vi "SETTINGS.vi"() -> ()   [LabVIEW 2021]
uses:
  Control 1.ctl
  ENNUM CONSTANT.ctl
  Control 4.ctl
  <vilib>/Utility/miscctls.llb/LVPointTypeDef.ctl
  SETTING CLOSE GLOBEL VARIABLE.vi
  <vilib>/Utility/config.llb/Write Key (String).vi
  <vilib>/Utility/config.llb/Write Key (Double).vi
  <vilib>/Utility/config.llb/NI_LVConfig.lvlib
panel:
  in  "Copy to alll":bool
  in  "ENTER":bool
  in  "PASS KEY":string
  in  "TIME DELAY":dbl
  in  "RETEST":bool
  out "String":string
  in  "VISA resource name":refnum<visa-resource-name>="COM5"
  in  "SAVE":bool
  in  "TOL 10":dbl
  in  "CH 10":dbl
  in  "TOL 9":dbl
  in  "CH 9":dbl
  in  "TOL 8":dbl
  in  "CH 8":dbl
  in  "TOL 7":dbl
  in  "CH 7":dbl
  in  "TOL 6":dbl
  in  "CH 6":dbl
  in  "TOL 5":dbl
  in  "CH 5":dbl
  in  "TOL 4":dbl
  in  "CH 4":dbl
  in  "TOL 3":dbl
  in  "CH 3":dbl
  in  "TOL 2":dbl
  in  "CH 2":dbl
  in  "TOL 1":dbl
  in  "CH 1":dbl
  in  "Combo Box":string(combo)
  in  "Home 2":T1
  # "EOL TEST BENCH FOR THERMISTOR"
  # "NOMINAL & TOLERANCE VALUES"
  # "MODE"
  # "DEVICE CONFIGURATION"
  # "k Ohm"
  # "Channel 1"
  # "%"
  # "REFERENCE RESISTANCE VALUE (CH 5)"
  # "COM PORT"
  # "k Ohm"
  # "Channel 2"
  # "%"
  # "k Ohm"
  # "Channel 3"
  # "k Ohm"
  # "%"
  # "Channel 4"
  # "k Ohm"
  # "%"
  # "Channel 5"
  # "k Ohm"
  # "%"
  # "THERMAL TIME DELAY"
  # "k Ohm"
  # "Channel 6"
  # "%"
  # "Sec"
  # "RETEST"
  # "k Ohm"
  # "Channel 7"
  # "%"
  # "k Ohm"
  # "Channel 8"
  # "%"
  # "AUTHENTICATION KEY"
  # "Channel 9"
  # "k Ohm"
  # "%"
  # "k Ohm"
  # "Channel 10"
  # "%"
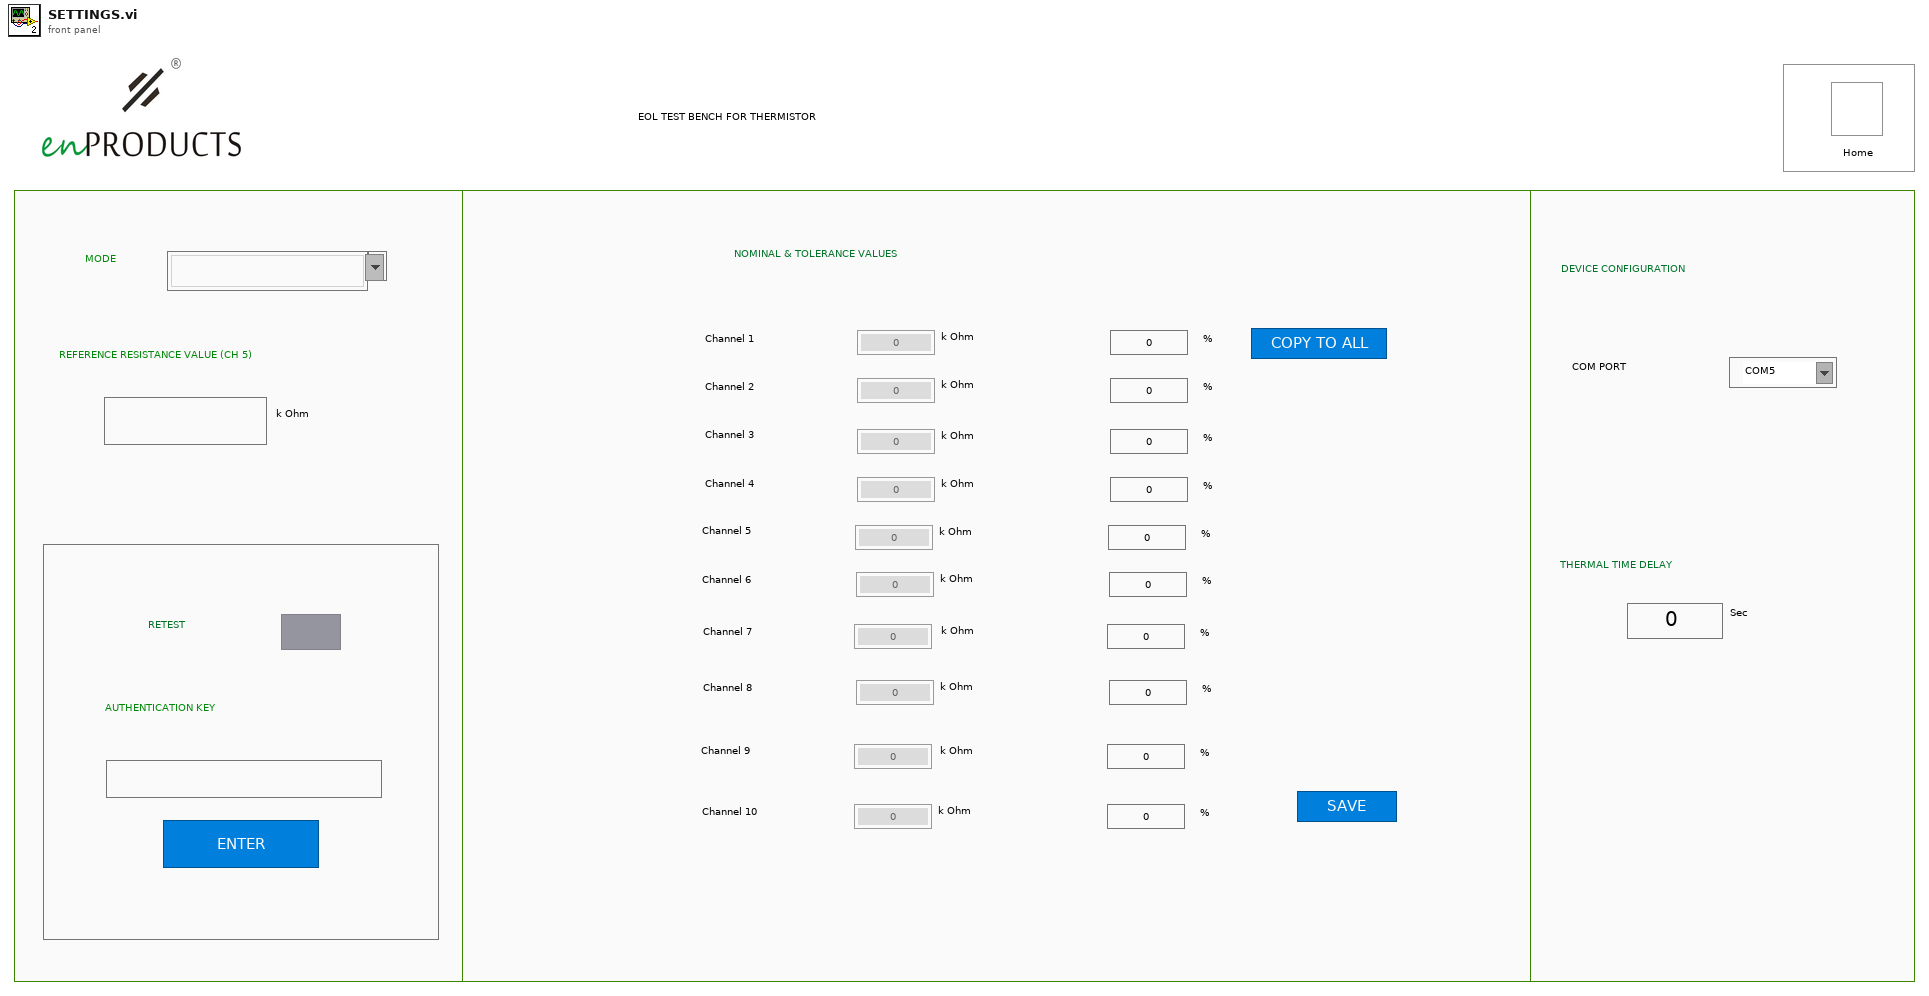
[diagram p1: front panel]
types:
  T1 = typedef "Control 1.ctl" = bool
  T2 = typedef "LVPointTypeDef.ctl" = cluster{"Horizontal":i16, "Vertical":i16}
  T3 = typedef "Control 4.ctl" = cluster{"VISA resource name":refnum<visa-resource-name>, "MODE":string, "PP 1":i32, "PP 2":i32, "PP 3":i32, "PP 4":i32, "PP 5":i32, "PP 6":i32, "PP 7":i32, "PP 8":i32, "PP 9":i32, "PP 10":i32, "CH  PASS  1":bool, "CH  PASS 2":bool, "CH  PASS 3":bool, "CH  PASS 4":bool, "CH  PASS 5":bool, "CH  PASS 6":bool, "CH  PASS 7":bool, "CH  PASS 8":bool, "CH  PASS 9":bool, "CH  PASS 10":bool, "CH  FAIL 1":bool, "CH  FAIL 2":bool, "CH  FAIL 3":bool, "CH  FAIL 4":bool, "CH  FAIL 5":bool, "CH  FAIL 6":bool, "CH  FAIL 7":bool, "CH  FAIL 8":bool, "CH  FAIL 9":bool, "CH  FAIL 10":bool, "RES VALUE 1":dbl, "RES VALUE 2":dbl, "RES VALUE 3":dbl, "RES VALUE 4":dbl, "RES VALUE 5":dbl, "RES VALUE 6":dbl, "RES VALUE 7":dbl, "RES VALUE 8":dbl, "RES VALUE 9":dbl, "RES VALUE 10":dbl, "SET VALUE 1":dbl, "SET VALUE 2":dbl, "SET VALUE 3":dbl, "SET VALUE 4":dbl, "SET VALUE 5":dbl, "SET VALUE 6":dbl, "SET VALUE 7":dbl, "SET VALUE 8":dbl, "SET VALUE 9":dbl, "SET VALUE 10":dbl, "TOL 1":dbl, "TOL 2":dbl, "TOL 3":dbl, "TOL 4":dbl, "TOL 5":dbl, "TOL 6":dbl, "TOL 7":dbl, "TOL 8":dbl, "TOL 9":dbl, "TOL 10":dbl, "START BIT":i32, "CH1 MIN TOL":dbl, "CH2 MIN TOL ":dbl, "CH3 MIN TOL ":dbl, "CH4 MIN TOL ":dbl, "CH5 MIN TOL ":dbl, "CH6 MIN TOL ":dbl, "CH7 MIN TOL  ":dbl, "CH8 MIN TOL  ":dbl, "CH9 MIN TOL   ":dbl, "CH10 MIN TOL   ":dbl, "CH1 MAX TOL ":dbl, "CH2 MAX TOL  ":dbl, "CH3 MAX TOL  ":dbl, "CH4 MAX TOL ":dbl, "CH5 MAX TOL  ":dbl, "CH6 MAX TOL  ":dbl, "CH7 MAX TOL   ":dbl, "CH8 MAX TOL  ":dbl, "CH9 MAX TOL    ":dbl, "CH10 MAX TOL   ":dbl}
  T4 = typedef "ENNUM CONSTANT.ctl" = enum16{"TIMEOUT", "INITIALIZE", "CONFIG READ", "CONFIG WRITE"}
  T5 = enum8{"Enabled", "Disabled", "Disabled and Grayed Out"}
  T6 = typedef "NI_LVConfig.lvlib/Config Data RefNum.ctl" = refnum<k1>
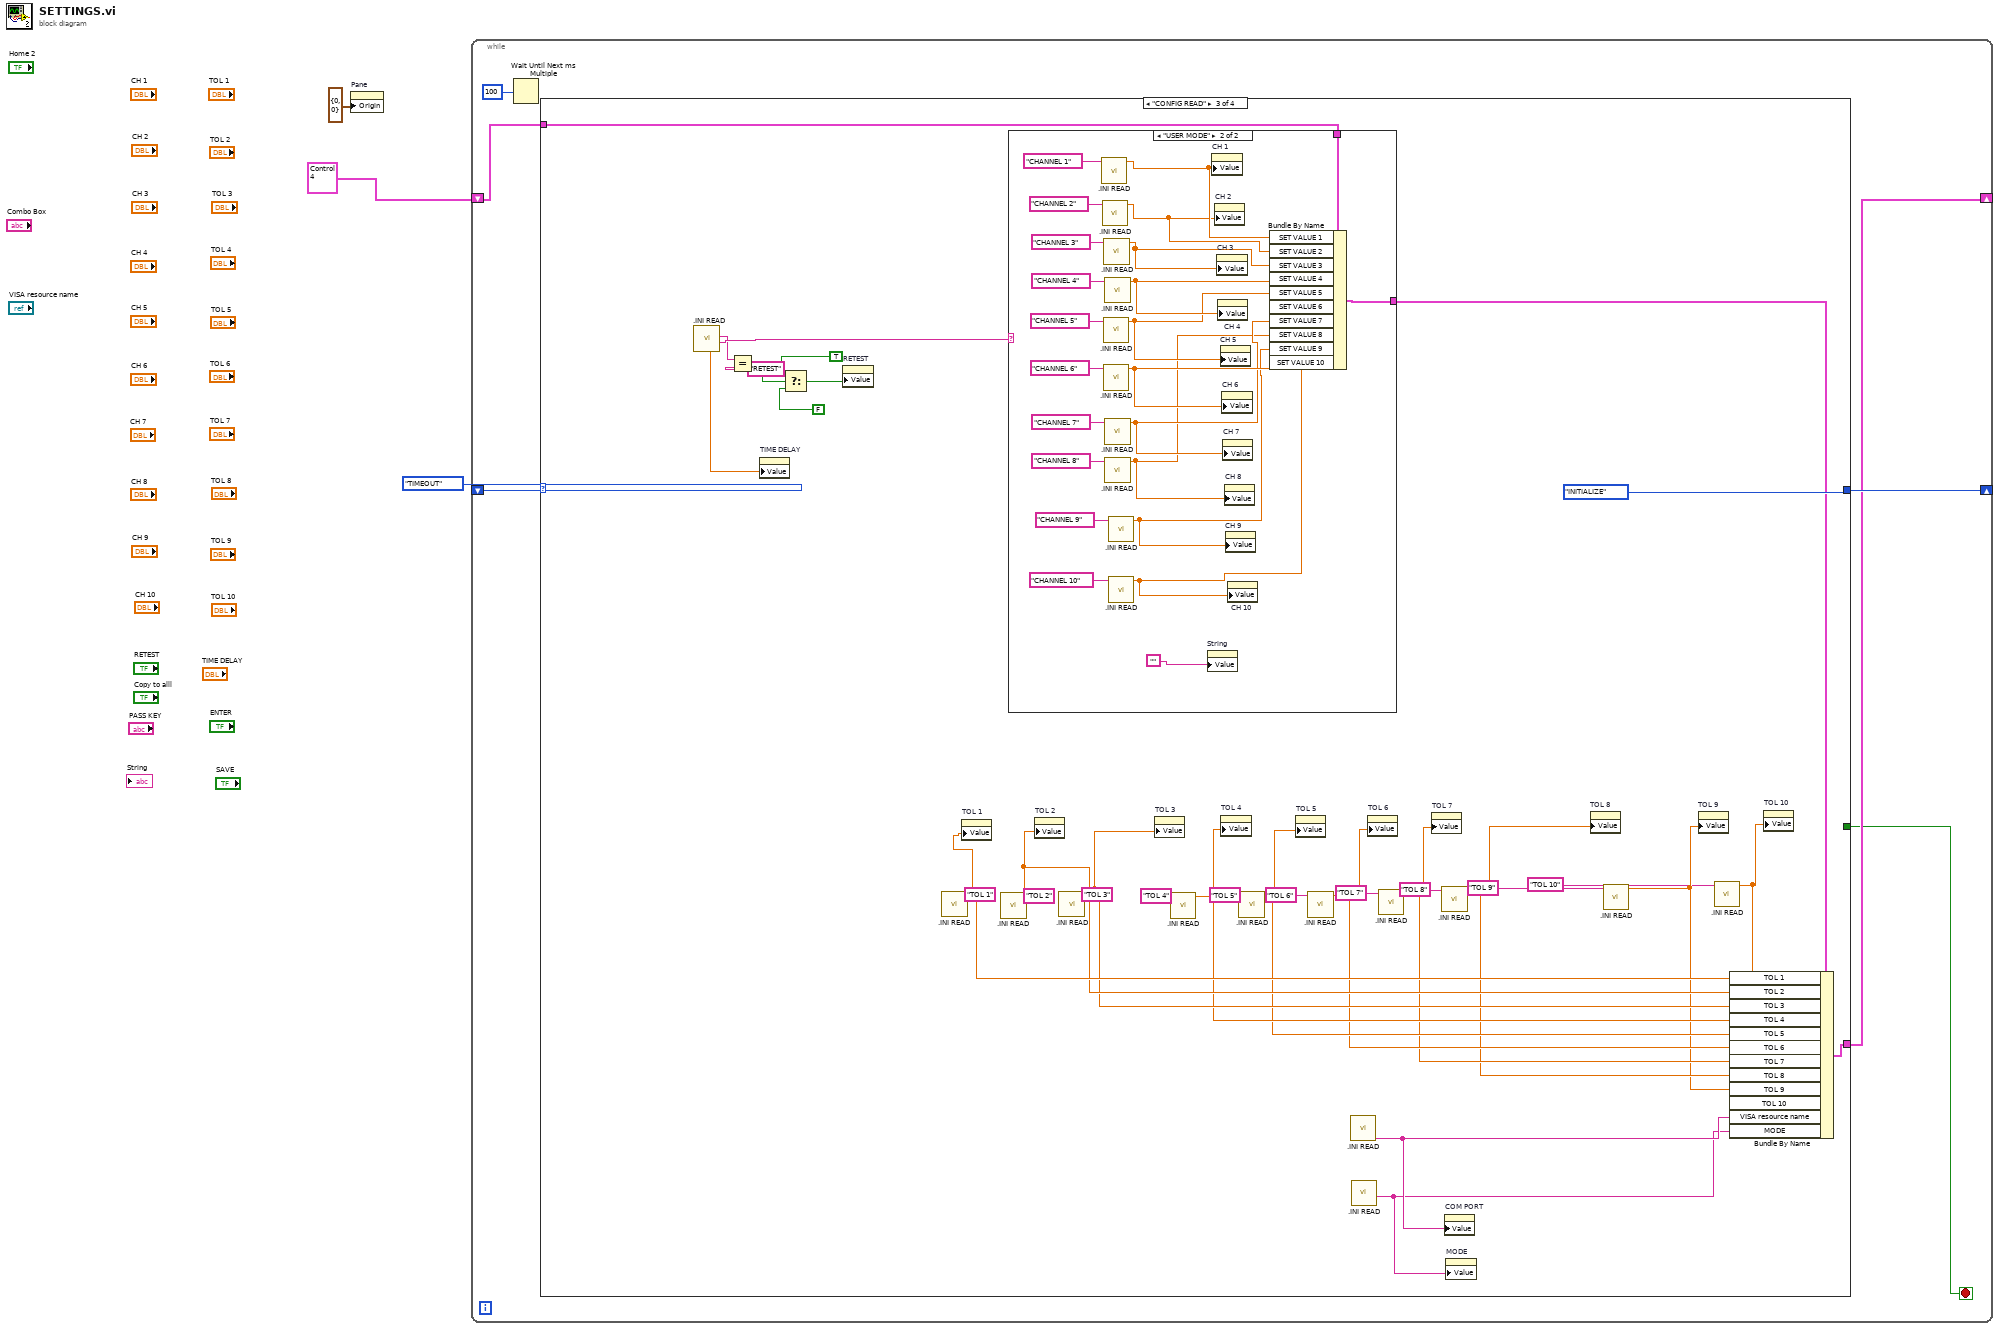
[diagram p0: block diagram]
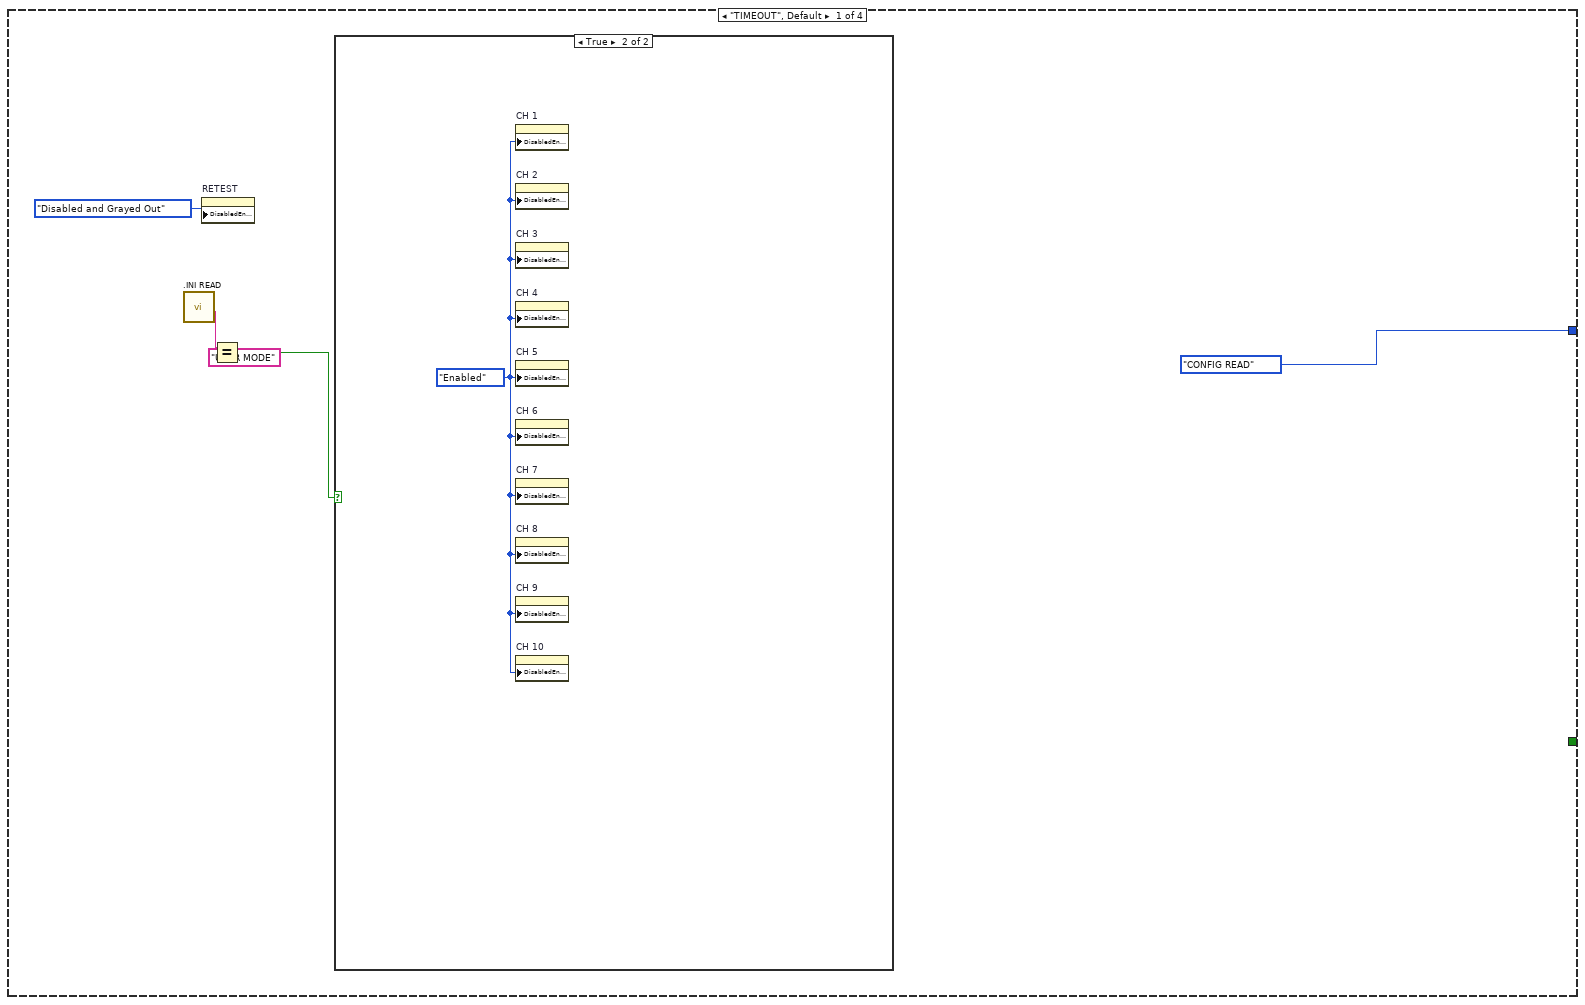
[diagram p2: hidden frame]
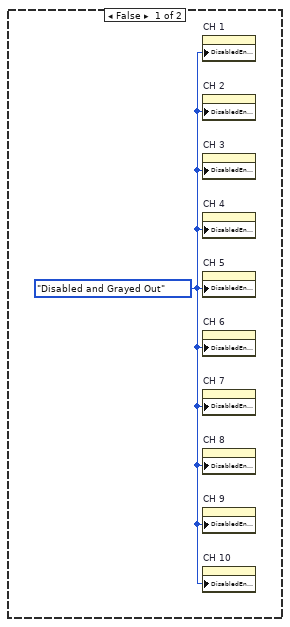
[diagram p3: hidden frame]
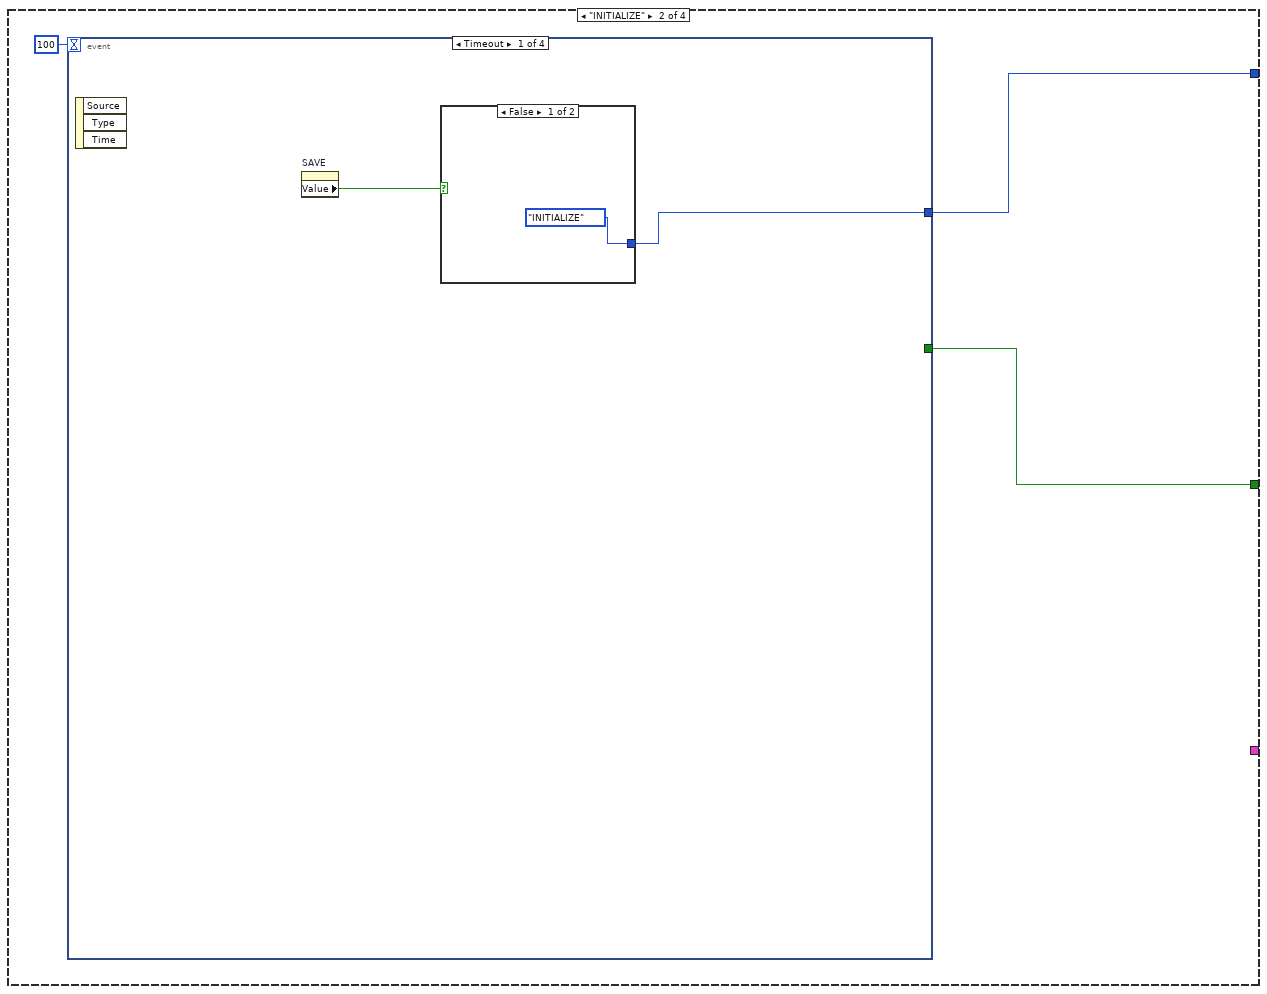
[diagram p4: hidden frame]
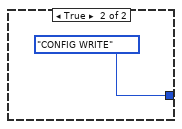
[diagram p5: hidden frame]
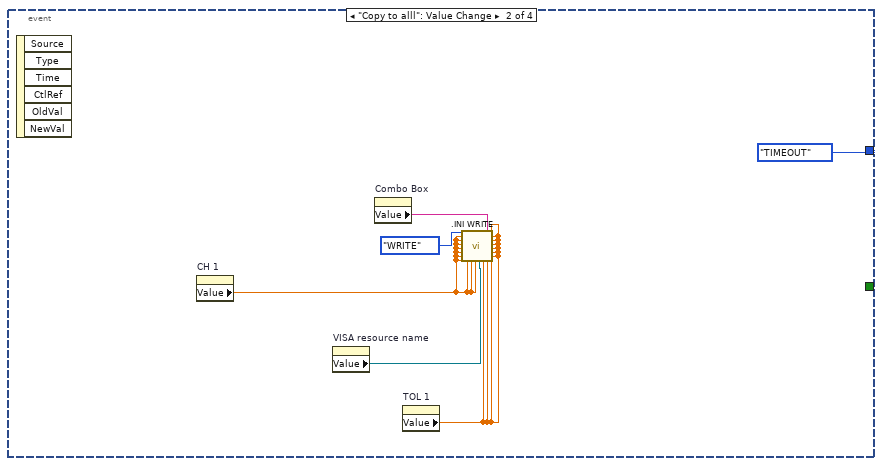
[diagram p6: hidden frame]
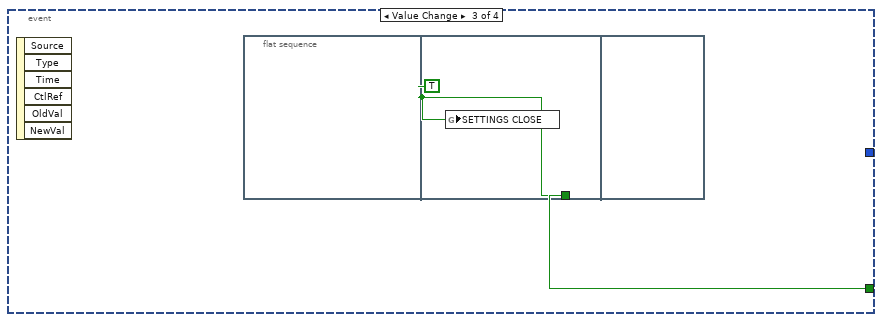
[diagram p7: hidden frame]
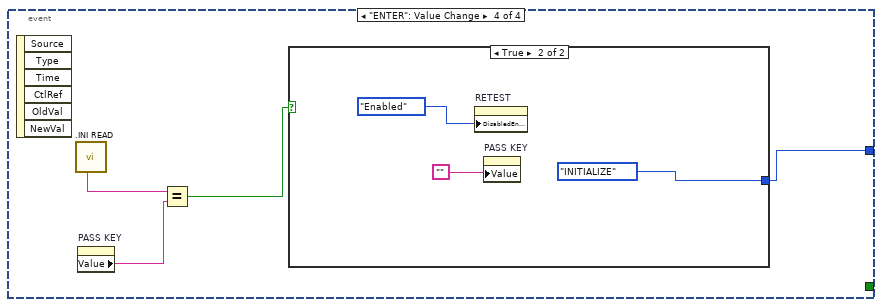
[diagram p8: hidden frame]
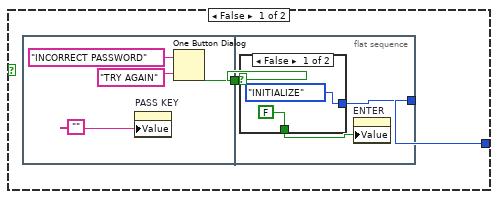
[diagram p9: hidden frame]
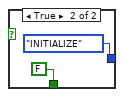
[diagram p10: hidden frame]
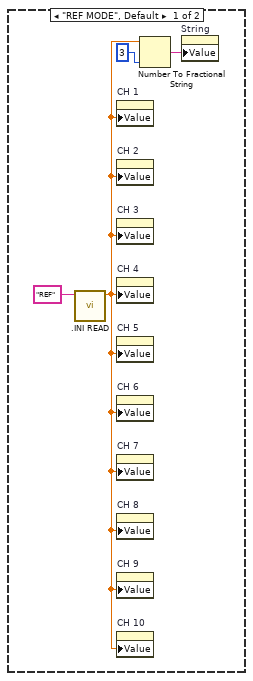
[diagram p11: hidden frame]
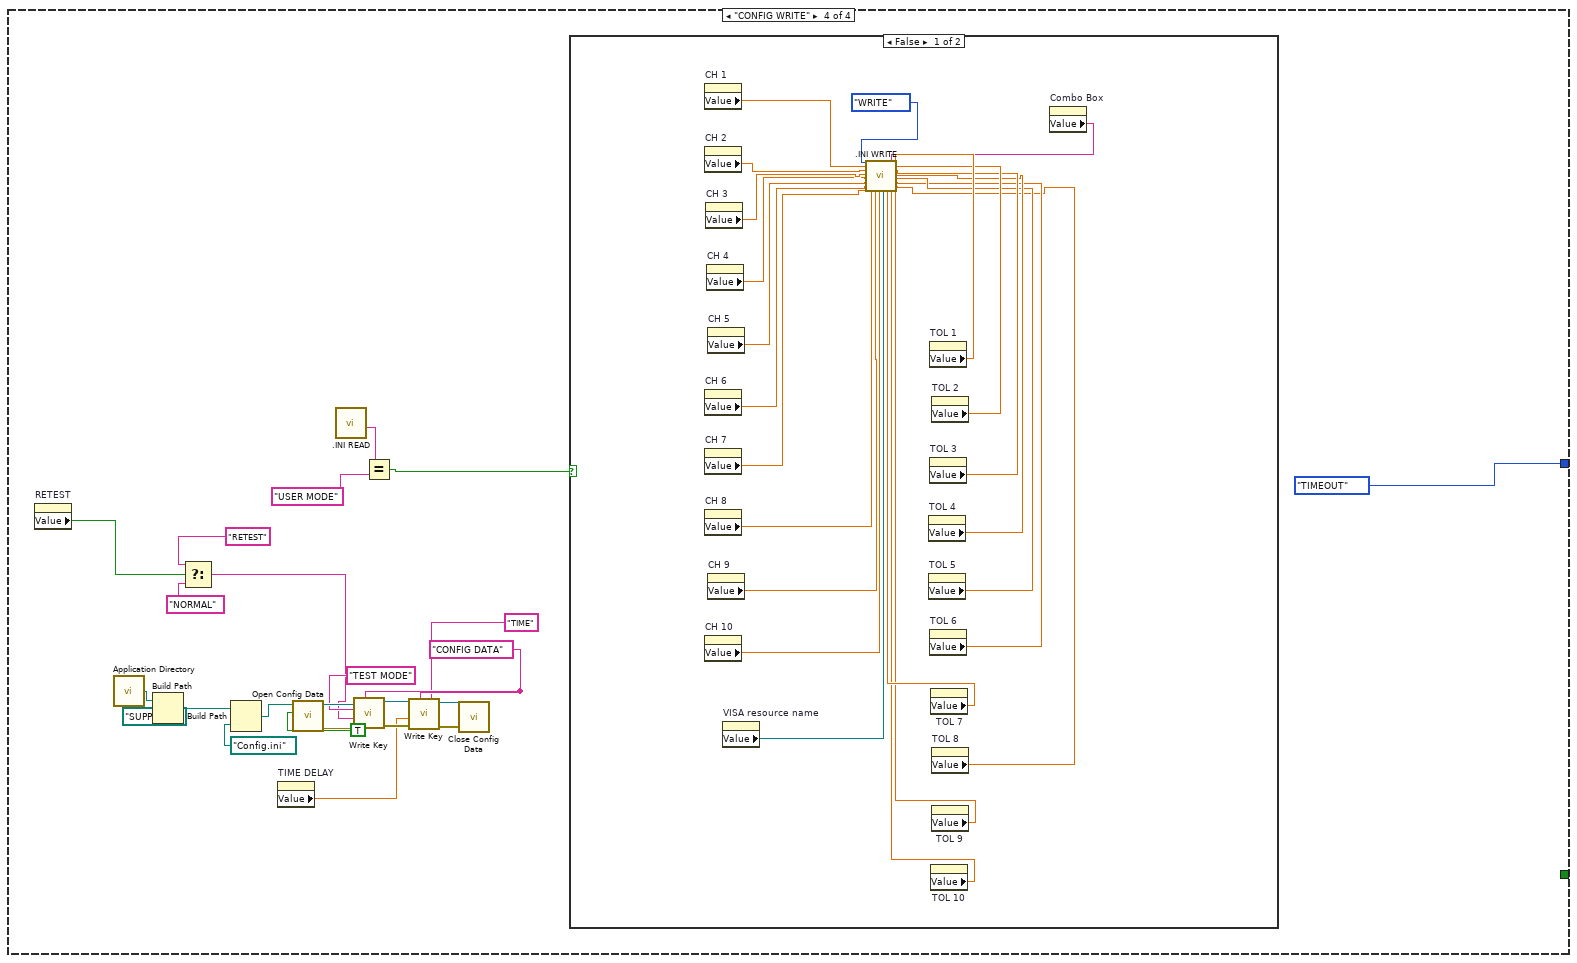
[diagram p12: hidden frame]
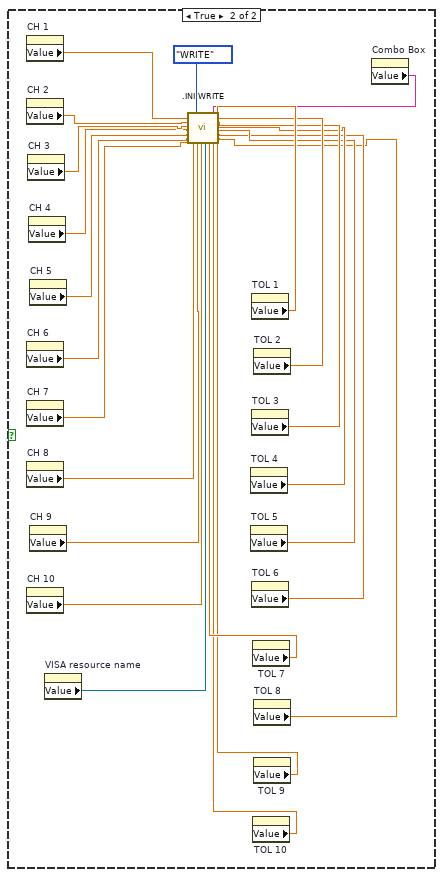
[diagram p13: hidden frame]
diagram:
  n1 = property on="Pane" class="Pane"("Origin"=T2 {"Horizontal"=0, "Vertical"=0}) -> ()  [unwired: 2 in, 2 out]
  n2 = while {
    shift-right: [w8] -> _
    shift-left: ENNUM_CONSTANT."TIMEOUT" -> [w9]
    shift-right: [w5] -> _
    shift-left: T3 {"VISA resource name"="COM5", "MODE"="", "PP 1"=0, "PP 2"=0, "PP 3"=0, "PP 4"=0, "PP 5"=0, "PP 6"=0, "PP 7"=0, "PP 8"=0, "PP 9"=0, "PP 10"=0, "CH  PASS  1"=FALSE, "CH  PASS 2"=FALSE, "CH  PASS 3"=FALSE, "CH  PASS 4"=FALSE, "CH  PASS 5"=FALSE, "CH  PASS 6"=FALSE, "CH  PASS 7"=FALSE, "CH  PASS 8"=FALSE, "CH  PASS 9"=FALSE, "CH  PASS 10"=FALSE, "CH  FAIL 1"=FALSE, "CH  FAIL 2"=FALSE, "CH  FAIL 3"=FALSE, "CH  FAIL 4"=FALSE, "CH  FAIL 5"=FALSE, "CH  FAIL 6"=FALSE, "CH  FAIL 7"=FALSE, "CH  FAIL 8"=FALSE, "CH  FAIL 9"=FALSE, "CH  FAIL 10"=FALSE, "RES VALUE 1"=0.0, "RES VALUE 2"=0.0, "RES VALUE 3"=0.0, "RES VALUE 4"=0.0, "RES VALUE 5"=0.0, "RES VALUE 6"=0.0, "RES VALUE 7"=0.0, "RES VALUE 8"=0.0, "RES VALUE 9"=0.0, "RES VALUE 10"=0.0, "SET VALUE 1"=0.0, "SET VALUE 2"=0.0, "SET VALUE 3"=0.0, "SET VALUE 4"=0.0, "SET VALUE 5"=0.0, "SET VALUE 6"=0.0, "SET VALUE 7"=0.0, "SET VALUE 8"=0.0, "SET VALUE 9"=0.0, "SET VALUE 10"=0.0, "TOL 1"=0.0, "TOL 2"=0.0, "TOL 3"=0.0, "TOL 4"=0.0, "TOL 5"=0.0, "TOL 6"=0.0, "TOL 7"=0.0, "TOL 8"=0.0, "TOL 9"=0.0, "TOL 10"=0.0, "START BIT"=0, "CH1 MIN TOL"=0.0, "CH2 MIN TOL "=0.0, "CH3 MIN TOL "=0.0, "CH4 MIN TOL "=0.0, "CH5 MIN TOL "=0.0, "CH6 MIN TOL "=0.0, "CH7 MIN TOL  "=0.0, "CH8 MIN TOL  "=0.0, "CH9 MIN TOL   "=0.0, "CH10 MIN TOL   "=0.0, "CH1 MAX TOL "=0.0, "CH2 MAX TOL  "=0.0, "CH3 MAX TOL  "=0.0, "CH4 MAX TOL "=0.0, "CH5 MAX TOL  "=0.0, "CH6 MAX TOL  "=0.0, "CH7 MAX TOL   "=0.0, "CH8 MAX TOL  "=0.0, "CH9 MAX TOL    "=0.0, "CH10 MAX TOL   "=0.0} -> [w6]
    stop <- w4 stop-if-true
    n3 = Wait Until Next ms Multiple(millisecond multiple=u32 100) -> ()  [unwired: 1 out]
    n4 = case shown="\"CONFIG READ\"" w9 {
      tunnel: [ENNUM_CONSTANT."CONFIG READ" w17 ENNUM_CONSTANT."INITIALIZE" ENNUM_CONSTANT."TIMEOUT"] -> w8
      tunnel: w6 -> [_ _ w60 _]
      tunnel: [_ _ w61 _] -> w5
      tunnel: [_ w18 _ _] -> w4
      frame "TIMEOUT", Default {
        n5 = call ".INI READ.vi"() -> ("MODE"=w13:string)  [unwired: 5 in, 6 out]
        n6 = property on="RETEST" class="Bool (strict)"("DisabledEnum"=T5."Disabled and Grayed Out" ("Disabled")) -> ()  [unwired: 2 in, 2 out]
        n7 = Equal?(x=w13, y="USER MODE") -> (x = y?=w11:bool)
        n8 = case shown="True" w11 {
          frame False {
            w15 = T5."Disabled and Grayed Out" ("Disabled")
            n9 = property on="CH 1" class="DigNum (strict)"("DisabledEnum"=w15) -> ()  [unwired: 2 in, 2 out]
            n10 = property on="CH 2" class="DigNum (strict)"("DisabledEnum"=w15) -> ()  [unwired: 2 in, 2 out]
            n11 = property on="CH 3" class="DigNum (strict)"("DisabledEnum"=w15) -> ()  [unwired: 2 in, 2 out]
            n12 = property on="CH 4" class="DigNum (strict)"("DisabledEnum"=w15) -> ()  [unwired: 2 in, 2 out]
            n13 = property on="CH 5" class="DigNum (strict)"("DisabledEnum"=w15) -> ()  [unwired: 2 in, 2 out]
            n14 = property on="CH 6" class="DigNum (strict)"("DisabledEnum"=w15) -> ()  [unwired: 2 in, 2 out]
            n15 = property on="CH 7" class="DigNum (strict)"("DisabledEnum"=w15) -> ()  [unwired: 2 in, 2 out]
            n16 = property on="CH 8" class="DigNum (strict)"("DisabledEnum"=w15) -> ()  [unwired: 2 in, 2 out]
            n17 = property on="CH 9" class="DigNum (strict)"("DisabledEnum"=w15) -> ()  [unwired: 2 in, 2 out]
            n18 = property on="CH 10" class="DigNum (strict)"("DisabledEnum"=w15) -> ()  [unwired: 2 in, 2 out]
          }
          frame True {
            w16 = T5."Enabled" ("Disabled")
            n19 = property on="CH 1" class="DigNum (strict)"("DisabledEnum"=w16) -> ()  [unwired: 2 in, 2 out]
            n20 = property on="CH 2" class="DigNum (strict)"("DisabledEnum"=w16) -> ()  [unwired: 2 in, 2 out]
            n21 = property on="CH 3" class="DigNum (strict)"("DisabledEnum"=w16) -> ()  [unwired: 2 in, 2 out]
            n22 = property on="CH 4" class="DigNum (strict)"("DisabledEnum"=w16) -> ()  [unwired: 2 in, 2 out]
            n23 = property on="CH 5" class="DigNum (strict)"("DisabledEnum"=w16) -> ()  [unwired: 2 in, 2 out]
            n24 = property on="CH 6" class="DigNum (strict)"("DisabledEnum"=w16) -> ()  [unwired: 2 in, 2 out]
            n25 = property on="CH 7" class="DigNum (strict)"("DisabledEnum"=w16) -> ()  [unwired: 2 in, 2 out]
            n26 = property on="CH 8" class="DigNum (strict)"("DisabledEnum"=w16) -> ()  [unwired: 2 in, 2 out]
            n27 = property on="CH 9" class="DigNum (strict)"("DisabledEnum"=w16) -> ()  [unwired: 2 in, 2 out]
            n28 = property on="CH 10" class="DigNum (strict)"("DisabledEnum"=w16) -> ()  [unwired: 2 in, 2 out]
          }
        }
      }
      frame "INITIALIZE" {
        n29 = event shown="[0] Timeout" {
          selector: _ -> [_ _ _ _]
          dyn-events: _ -> [_ _ _ _]
          timeout: 100 -> [_ _ _ _]
          tunnel: [_ _ w30 _] -> w18
          tunnel: [w20 ENNUM_CONSTANT."TIMEOUT" _ w32] -> w17
          event Timeout {
            n30 = event-data() -> ()  [unwired: 1 in, 3 out]
            n31 = property on="SAVE" class="Bool (strict)"() -> ("Value"=w21:bool)  [unwired: 2 in, 2 out]
            n32 = case shown="False" w21 {
              tunnel: [ENNUM_CONSTANT."INITIALIZE" ENNUM_CONSTANT."CONFIG WRITE"] -> w20
              frame False {
              }
              frame True {
              }
            }
          }
          event "Copy to alll": Value Change {
            n33 = event-data() -> ()  [unwired: 1 in, 6 out]
            n34 = property on="CH 1" class="DigNum (strict)"() -> ("Value"=w25:dbl)  [unwired: 2 in, 2 out]
            n35 = property on="VISA resource name" class="VISAName"() -> ("Value"=w27:refnum<visa-resource-name>)  [unwired: 2 in, 2 out]
            n36 = property on="Combo Box" class="CmbBox"() -> ("Value"=w28:string)  [unwired: 2 in, 2 out]
            n37 = property on="TOL 1" class="DigNum (strict)"() -> ("Value"=w24:dbl)  [unwired: 2 in, 2 out]
            n38 = call ".INI WRITE.vi"("Enum"=enum16{"READ", "WRITE"}."WRITE", "CH 1"=w25, "CH 2"=w25, "CH 3"=w25, "CH 4"=w25, "CH 5"=w25, "CH 6"=w25, "CH 7"=w25, "CH 8"=w25, "CH 9"=w25, "CH 10"=w25, "COM"=w27, "TOL 7"=w24, "MODE"=w28, "TOL 10"=w24, "TOL 1"=w24, "TOL 2"=w24, "TOL 3"=w24, "TOL 4"=w24, "TOL 5"=w24, "TOL 6"=w24, "TOL 8"=w24, "TOL 9"=w24) -> ()  [unwired: 5 in]
          }
          event Value Change {
            n39 = event-data() -> ()  [unwired: 1 in, 6 out]
            n40 = flat-sequence {
              tunnel: [w31] -> w30
              frame #0 {
              }
              frame #1 {
                w31 = TRUE
                n41 = global write "SETTING CLOSE GLOBEL VARIABLE.vi" "SETTINGS CLOSE"(w31) -> ()
              }
              frame #2 {
              }
            }
          }
          event "ENTER": Value Change {
            n42 = event-data() -> ()  [unwired: 1 in, 6 out]
            n43 = call ".INI READ.vi"() -> ("AUTH KEY"=w35:string)  [unwired: 5 in, 6 out]
            n44 = property on="PASS KEY" class="Str"() -> ("Value"=w34:string)  [unwired: 2 in, 2 out]
            n45 = Equal?(x=w35, y=w34) -> (x = y?=w33:bool)
            n46 = case shown="True" w33 {
              tunnel: [w36 ENNUM_CONSTANT."INITIALIZE"] -> w32
              frame False {
                n47 = flat-sequence {
                  tunnel: [w38] -> w37
                  tunnel: w37 -> [w44]
                  tunnel: [w43] -> w36
                  frame #0 {
                    n48 = property on="PASS KEY" class="Str"("Value"="") -> ()  [unwired: 2 in, 2 out]
                    n49 = One Button Dialog(message="INCORRECT PASSWORD", button name ("OK")="TRY AGAIN") -> (true=w38:bool)
                  }
                  frame #1 {
                    n50 = case shown="False" w44 {
                      tunnel: [ENNUM_CONSTANT."INITIALIZE" ENNUM_CONSTANT."INITIALIZE"] -> w43
                      tunnel: [FALSE FALSE] -> w42
                      frame False {
                      }
                      frame True {
                      }
                    }
                    n51 = property on="ENTER" class="Bool (strict)"("Value"=w42) -> ()  [unwired: 2 in, 2 out]
                  }
                }
              }
              frame True {
                n52 = property on="RETEST" class="Bool (strict)"("DisabledEnum"=T5."Enabled" ("Disabled")) -> ()  [unwired: 2 in, 2 out]
                n53 = property on="PASS KEY" class="Str"("Value"="") -> ()  [unwired: 2 in, 2 out]
              }
            }
          }
        }
      }
      frame "CONFIG READ" {
        n54 = call ".INI READ.vi"() -> ("MODE"=w62:string, "TEST MODE"=w53:string, "TIME"=w52:dbl)  [unwired: 5 in, 4 out]
        n55 = Equal?(x=w53, y="RETEST") -> (x = y?=w57:bool)
        n56 = property on="TIME DELAY" class="DigNum (strict)"("Value"=w52) -> ()  [unwired: 2 in, 2 out]
        n57 = Select(t=TRUE, s=w57, f=FALSE) -> (s? t:f=w54:bool)
        n58 = property on="RETEST" class="Bool (strict)"("Value"=w54) -> ()  [unwired: 2 in, 2 out]
        n59 = call ".INI READ.vi"("KEY"="TOL 1") -> ("OUT"=w83:dbl)  [unwired: 4 in, 6 out]
        n60 = property on="TOL 1" class="DigNum (strict)"("Value"=w83) -> ()  [unwired: 2 in, 2 out]
        n61 = call ".INI READ.vi"("KEY"="TOL 2") -> ("OUT"=w80:dbl)  [unwired: 4 in, 6 out]
        n62 = case shown="\"USER MODE\"" w62 {
          tunnel: w60 -> [_ w92]
          tunnel: [_ w91] -> w59
          frame "REF MODE", Default {
            n63 = call ".INI READ.vi"("KEY"="REF") -> ("OUT"=w86:dbl)  [unwired: 4 in, 6 out]
            n64 = property on="CH 1" class="DigNum (strict)"("Value"=w86) -> ()  [unwired: 2 in, 2 out]
            n65 = property on="CH 2" class="DigNum (strict)"("Value"=w86) -> ()  [unwired: 2 in, 2 out]
            n66 = property on="CH 3" class="DigNum (strict)"("Value"=w86) -> ()  [unwired: 2 in, 2 out]
            n67 = property on="CH 4" class="DigNum (strict)"("Value"=w86) -> ()  [unwired: 2 in, 2 out]
            n68 = property on="CH 5" class="DigNum (strict)"("Value"=w86) -> ()  [unwired: 2 in, 2 out]
            n69 = property on="CH 6" class="DigNum (strict)"("Value"=w86) -> ()  [unwired: 2 in, 2 out]
            n70 = property on="CH 7" class="DigNum (strict)"("Value"=w86) -> ()  [unwired: 2 in, 2 out]
            n71 = property on="CH 8" class="DigNum (strict)"("Value"=w86) -> ()  [unwired: 2 in, 2 out]
            n72 = property on="CH 9" class="DigNum (strict)"("Value"=w86) -> ()  [unwired: 2 in, 2 out]
            n73 = property on="CH 10" class="DigNum (strict)"("Value"=w86) -> ()  [unwired: 2 in, 2 out]
            n74 = Number To Fractional String(number=w86, precision (6)=i16 3) -> (F-format string=w88:string)  [unwired: 2 in]
            n75 = property on="String" class="Str"("Value"=w88) -> ()  [unwired: 2 in, 2 out]
          }
          frame "USER MODE" {
            n76 = call ".INI READ.vi"("KEY"="CHANNEL 1") -> ("OUT"=w111:dbl)  [unwired: 4 in, 6 out]
            n77 = call ".INI READ.vi"("KEY"="CHANNEL 2") -> ("OUT"=w109:dbl)  [unwired: 4 in, 6 out]
            n78 = call ".INI READ.vi"("KEY"="CHANNEL 5") -> ("OUT"=w103:dbl)  [unwired: 4 in, 6 out]
            n79 = call ".INI READ.vi"("KEY"="CHANNEL 6") -> ("OUT"=w101:dbl)  [unwired: 4 in, 6 out]
            n80 = call ".INI READ.vi"("KEY"="CHANNEL 3") -> ("OUT"=w107:dbl)  [unwired: 4 in, 6 out]
            n81 = call ".INI READ.vi"("KEY"="CHANNEL 4") -> ("OUT"=w105:dbl)  [unwired: 4 in, 6 out]
            n82 = call ".INI READ.vi"("KEY"="CHANNEL 7") -> ("OUT"=w99:dbl)  [unwired: 4 in, 6 out]
            n83 = call ".INI READ.vi"("KEY"="CHANNEL 8") -> ("OUT"=w97:dbl)  [unwired: 4 in, 6 out]
            n84 = call ".INI READ.vi"("KEY"="CHANNEL 9") -> ("OUT"=w95:dbl)  [unwired: 4 in, 6 out]
            n85 = call ".INI READ.vi"("KEY"="CHANNEL 10") -> ("OUT"=w93:dbl)  [unwired: 4 in, 6 out]
            n86 = property on="String" class="Str"("Value"="") -> ()  [unwired: 2 in, 2 out]
            n87 = property on="CH 1" class="DigNum (strict)"("Value"=w111) -> ()  [unwired: 2 in, 2 out]
            n88 = property on="CH 2" class="DigNum (strict)"("Value"=w109) -> ()  [unwired: 2 in, 2 out]
            n89 = property on="CH 3" class="DigNum (strict)"("Value"=w107) -> ()  [unwired: 2 in, 2 out]
            n90 = property on="CH 4" class="DigNum (strict)"("Value"=w105) -> ()  [unwired: 2 in, 2 out]
            n91 = property on="CH 5" class="DigNum (strict)"("Value"=w103) -> ()  [unwired: 2 in, 2 out]
            n92 = property on="CH 6" class="DigNum (strict)"("Value"=w101) -> ()  [unwired: 2 in, 2 out]
            n93 = property on="CH 7" class="DigNum (strict)"("Value"=w99) -> ()  [unwired: 2 in, 2 out]
            n94 = property on="CH 8" class="DigNum (strict)"("Value"=w97) -> ()  [unwired: 2 in, 2 out]
            n95 = property on="CH 9" class="DigNum (strict)"("Value"=w95) -> ()  [unwired: 2 in, 2 out]
            n96 = property on="CH 10" class="DigNum (strict)"("Value"=w93) -> ()  [unwired: 2 in, 2 out]
            n97 = Bundle By Name(cluster=w92, "SET VALUE 1"=w111, "SET VALUE 2"=w109, "SET VALUE 3"=w107, "SET VALUE 4"=w105, "SET VALUE 5"=w103, "SET VALUE 6"=w101, "SET VALUE 7"=w99, "SET VALUE 8"=w97, "SET VALUE 9"=w95, "SET VALUE 10"=w93) -> (w91:T3)
          }
        }
        n98 = property on="TOL 2" class="DigNum (strict)"("Value"=w80) -> ()  [unwired: 2 in, 2 out]
        n99 = call ".INI READ.vi"("KEY"="TOL 3") -> ("OUT"=w79:dbl)  [unwired: 4 in, 6 out]
        n100 = property on="TOL 3" class="DigNum (strict)"("Value"=w79) -> ()  [unwired: 2 in, 2 out]
        n101 = call ".INI READ.vi"("KEY"="TOL 4") -> ("OUT"=w77:dbl)  [unwired: 4 in, 6 out]
        n102 = property on="TOL 4" class="DigNum (strict)"("Value"=w77) -> ()  [unwired: 2 in, 2 out]
        n103 = call ".INI READ.vi"("KEY"="TOL 5") -> ("OUT"=w75:dbl)  [unwired: 4 in, 6 out]
        n104 = property on="TOL 5" class="DigNum (strict)"("Value"=w75) -> ()  [unwired: 2 in, 2 out]
        n105 = call ".INI READ.vi"("KEY"="TOL 6") -> ("OUT"=w73:dbl)  [unwired: 4 in, 6 out]
        n106 = call ".INI READ.vi"() -> ("COM"=w64:string)  [unwired: 5 in, 6 out]
        n107 = call ".INI READ.vi"() -> ("MODE"=w63:string)  [unwired: 5 in, 6 out]
        n108 = property on="TOL 6" class="DigNum (strict)"("Value"=w73) -> ()  [unwired: 2 in, 2 out]
        n109 = call ".INI READ.vi"("KEY"="TOL 7") -> ("OUT"=w71:dbl)  [unwired: 4 in, 6 out]
        n110 = property on="TOL 7" class="DigNum (strict)"("Value"=w71) -> ()  [unwired: 2 in, 2 out]
        n111 = call ".INI READ.vi"("KEY"="TOL 8") -> ("OUT"=w69:dbl)  [unwired: 4 in, 6 out]
        n112 = property on="COM PORT" class="VISAName"("Value"=w64) -> ()  [unwired: 2 in, 2 out]
        n113 = property on="MODE" class="CmbBox"("Value"=w63) -> ()  [unwired: 2 in, 2 out]
        n114 = property on="TOL 8" class="DigNum (strict)"("Value"=w69) -> ()  [unwired: 2 in, 2 out]
        n115 = call ".INI READ.vi"("KEY"="TOL 9") -> ("OUT"=w67:dbl)  [unwired: 4 in, 6 out]
        n116 = property on="TOL 9" class="DigNum (strict)"("Value"=w67) -> ()  [unwired: 2 in, 2 out]
        n117 = call ".INI READ.vi"("KEY"="TOL 10") -> ("OUT"=w65:dbl)  [unwired: 4 in, 6 out]
        n118 = Bundle By Name(cluster=w59, "TOL 1"=w83, "TOL 2"=w80, "TOL 3"=w79, "TOL 4"=w77, "TOL 5"=w75, "TOL 6"=w73, "TOL 7"=w71, "TOL 8"=w69, "TOL 9"=w67, "TOL 10"=w65, "VISA resource name"=w64, "MODE"=w63) -> (w61:T3)
        n119 = property on="TOL 10" class="DigNum (strict)"("Value"=w65) -> ()  [unwired: 2 in, 2 out]
      }
      frame "CONFIG WRITE" {
        w115 = "CONFIG DATA" ("section")
        n120 = property on="RETEST" class="Bool (strict)"() -> ("Value"=w123:bool)  [unwired: 2 in, 2 out]
        n121 = call <vilib>:"Application Directory.vi"() -> ("Application Directory"=w131:path)
        n122 = Build Path(base path=w131, name or relative path=path "SUPPORT") -> (appended path=w132:path)
        n123 = Select(t="RETEST", s=w123, f="NORMAL") -> (s? t:f=w120:string)
        n124 = Build Path(base path=w132, name or relative path=path "Config.ini") -> (appended path=w128:path)
        n125 = property on="TIME DELAY" class="DigNum (strict)"() -> ("Value"=w113:dbl)  [unwired: 2 in, 2 out]
        n126 = call <vilib>:"Open Config Data.vi"("create file if necessary (T)"=TRUE, "configuration file path"=w128) -> ("error out"=w124:errorcluster, "refnum"=w126:T6)  [unwired: 7 in, 1 out]
        n127 = call ".INI READ.vi"() -> ("MODE"=w135:string)  [unwired: 5 in, 6 out]
        n128 = call-poly <vilib>:"Write Key.vi"("section"=w115, "error in (no error)"=w124, "value"=w120, "key"="TEST MODE", "refnum"=w126) -> ("error out"=w116:errorcluster, "refnum out"=w117:T6)  [unwired: 4 in, 1 out]
        n129 = Equal?(x=w135, y="USER MODE") -> (x = y?=w134:bool)
        n130 = call-poly <vilib>:"Write Key.vi"("section"=w115, "error in (no error)"=w116, "value"=w113, "key"="TIME", "refnum"=w117) -> ("error out"=w119:errorcluster, "refnum out"=w118:T6)  [unwired: 4 in, 1 out]
        n131 = call <vilib>:"Close Config Data.vi"("error in (no error)"=w119, "refnum"=w118) -> ()  [unwired: 8 in, 2 out]
        n132 = case shown="False" w134 {
          frame False {
            n133 = property on="CH 1" class="DigNum (strict)"() -> ("Value"=w159:dbl)  [unwired: 2 in, 2 out]
            n134 = property on="CH 2" class="DigNum (strict)"() -> ("Value"=w158:dbl)  [unwired: 2 in, 2 out]
            n135 = property on="CH 6" class="DigNum (strict)"() -> ("Value"=w154:dbl)  [unwired: 2 in, 2 out]
            n136 = property on="CH 7" class="DigNum (strict)"() -> ("Value"=w153:dbl)  [unwired: 2 in, 2 out]
            n137 = property on="CH 8" class="DigNum (strict)"() -> ("Value"=w152:dbl)  [unwired: 2 in, 2 out]
            n138 = property on="CH 10" class="DigNum (strict)"() -> ("Value"=w150:dbl)  [unwired: 2 in, 2 out]
            n139 = property on="CH 3" class="DigNum (strict)"() -> ("Value"=w157:dbl)  [unwired: 2 in, 2 out]
            n140 = property on="CH 4" class="DigNum (strict)"() -> ("Value"=w156:dbl)  [unwired: 2 in, 2 out]
            n141 = property on="CH 5" class="DigNum (strict)"() -> ("Value"=w155:dbl)  [unwired: 2 in, 2 out]
            n142 = property on="CH 9" class="DigNum (strict)"() -> ("Value"=w151:dbl)  [unwired: 2 in, 2 out]
            n143 = property on="VISA resource name" class="VISAName"() -> ("Value"=w138:refnum<visa-resource-name>)  [unwired: 2 in, 2 out]
            n144 = property on="TOL 4" class="DigNum (strict)"() -> ("Value"=w146:dbl)  [unwired: 2 in, 2 out]
            n145 = property on="TOL 5" class="DigNum (strict)"() -> ("Value"=w145:dbl)  [unwired: 2 in, 2 out]
            n146 = property on="TOL 1" class="DigNum (strict)"() -> ("Value"=w149:dbl)  [unwired: 2 in, 2 out]
            n147 = property on="TOL 3" class="DigNum (strict)"() -> ("Value"=w147:dbl)  [unwired: 2 in, 2 out]
            n148 = property on="TOL 6" class="DigNum (strict)"() -> ("Value"=w144:dbl)  [unwired: 2 in, 2 out]
            n149 = property on="TOL 7" class="DigNum (strict)"() -> ("Value"=w143:dbl)  [unwired: 2 in, 2 out]
            n150 = property on="TOL 10" class="DigNum (strict)"() -> ("Value"=w140:dbl)  [unwired: 2 in, 2 out]
            n151 = property on="TOL 2" class="DigNum (strict)"() -> ("Value"=w148:dbl)  [unwired: 2 in, 2 out]
            n152 = property on="TOL 8" class="DigNum (strict)"() -> ("Value"=w142:dbl)  [unwired: 2 in, 2 out]
            n153 = property on="TOL 9" class="DigNum (strict)"() -> ("Value"=w141:dbl)  [unwired: 2 in, 2 out]
            n154 = property on="Combo Box" class="CmbBox"() -> ("Value"=w139:string)  [unwired: 2 in, 2 out]
            n155 = call ".INI WRITE.vi"("Enum"=enum16{"READ", "WRITE"}."WRITE", "CH 1"=w159, "CH 2"=w158, "CH 3"=w157, "CH 4"=w156, "CH 5"=w155, "CH 6"=w154, "CH 7"=w153, "CH 8"=w152, "CH 9"=w151, "CH 10"=w150, "COM"=w138, "TOL 7"=w143, "MODE"=w139, "TOL 10"=w140, "TOL 1"=w149, "TOL 2"=w148, "TOL 3"=w147, "TOL 4"=w146, "TOL 5"=w145, "TOL 6"=w144, "TOL 8"=w142, "TOL 9"=w141) -> ()  [unwired: 5 in]
          }
          frame True {
            n156 = property on="CH 1" class="DigNum (strict)"() -> ("Value"=w181:dbl)  [unwired: 2 in, 2 out]
            n157 = property on="CH 2" class="DigNum (strict)"() -> ("Value"=w180:dbl)  [unwired: 2 in, 2 out]
            n158 = property on="CH 6" class="DigNum (strict)"() -> ("Value"=w176:dbl)  [unwired: 2 in, 2 out]
            n159 = property on="CH 7" class="DigNum (strict)"() -> ("Value"=w175:dbl)  [unwired: 2 in, 2 out]
            n160 = property on="CH 8" class="DigNum (strict)"() -> ("Value"=w174:dbl)  [unwired: 2 in, 2 out]
            n161 = property on="CH 10" class="DigNum (strict)"() -> ("Value"=w172:dbl)  [unwired: 2 in, 2 out]
            n162 = property on="CH 3" class="DigNum (strict)"() -> ("Value"=w179:dbl)  [unwired: 2 in, 2 out]
            n163 = property on="CH 4" class="DigNum (strict)"() -> ("Value"=w178:dbl)  [unwired: 2 in, 2 out]
            n164 = property on="CH 5" class="DigNum (strict)"() -> ("Value"=w177:dbl)  [unwired: 2 in, 2 out]
            n165 = property on="CH 9" class="DigNum (strict)"() -> ("Value"=w173:dbl)  [unwired: 2 in, 2 out]
            n166 = property on="VISA resource name" class="VISAName"() -> ("Value"=w160:refnum<visa-resource-name>)  [unwired: 2 in, 2 out]
            n167 = property on="TOL 4" class="DigNum (strict)"() -> ("Value"=w168:dbl)  [unwired: 2 in, 2 out]
            n168 = property on="TOL 5" class="DigNum (strict)"() -> ("Value"=w167:dbl)  [unwired: 2 in, 2 out]
            n169 = property on="TOL 1" class="DigNum (strict)"() -> ("Value"=w171:dbl)  [unwired: 2 in, 2 out]
            n170 = property on="TOL 3" class="DigNum (strict)"() -> ("Value"=w169:dbl)  [unwired: 2 in, 2 out]
            n171 = property on="TOL 6" class="DigNum (strict)"() -> ("Value"=w166:dbl)  [unwired: 2 in, 2 out]
            n172 = property on="TOL 7" class="DigNum (strict)"() -> ("Value"=w165:dbl)  [unwired: 2 in, 2 out]
            n173 = property on="TOL 10" class="DigNum (strict)"() -> ("Value"=w162:dbl)  [unwired: 2 in, 2 out]
            n174 = property on="TOL 2" class="DigNum (strict)"() -> ("Value"=w170:dbl)  [unwired: 2 in, 2 out]
            n175 = property on="TOL 8" class="DigNum (strict)"() -> ("Value"=w164:dbl)  [unwired: 2 in, 2 out]
            n176 = property on="TOL 9" class="DigNum (strict)"() -> ("Value"=w163:dbl)  [unwired: 2 in, 2 out]
            n177 = property on="Combo Box" class="CmbBox"() -> ("Value"=w161:string)  [unwired: 2 in, 2 out]
            n178 = call ".INI WRITE.vi"("Enum"=enum16{"READ", "WRITE"}."WRITE", "CH 1"=w181, "CH 2"=w180, "CH 3"=w179, "CH 4"=w178, "CH 5"=w177, "CH 6"=w176, "CH 7"=w175, "CH 8"=w174, "CH 9"=w173, "CH 10"=w172, "COM"=w160, "TOL 7"=w165, "MODE"=w161, "TOL 10"=w162, "TOL 1"=w171, "TOL 2"=w170, "TOL 3"=w169, "TOL 4"=w168, "TOL 5"=w167, "TOL 6"=w166, "TOL 8"=w164, "TOL 9"=w163) -> ()  [unwired: 5 in]
          }
        }
      }
    }
  }
